vi "Load Command.vi"(8 "error in (no error)":errorcluster, 9 "Front (T) Back (F)":bool, 10 "Command In":refnum<class "Command.lvclass">, 11 "Command Handler in":refnum<class "Command Handler.lvclass">) -> (0 "error out":errorcluster, 3 "Command Handler out":refnum<class "Command Handler.lvclass">)   [LabVIEW 2017, in "Command Handler.lvlib" / "Command Handler.lvclass"]
uses:
  Command Handler.lvclass
  Command Parents/Command.lvclass
  Command Handler.lvclass/Command Handler.ctl
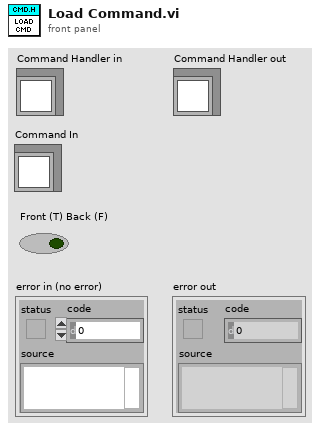
[diagram p1: front panel]
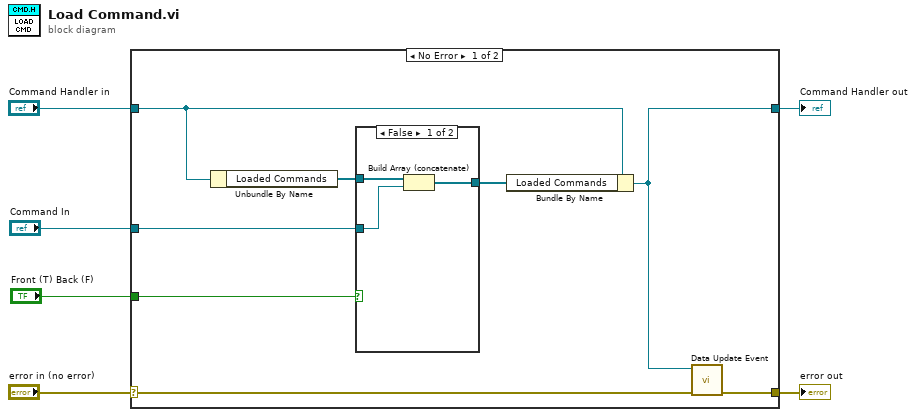
[diagram p0: block diagram]
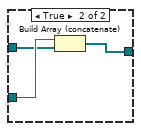
[diagram p2: hidden frame]
diagram:
  n1 = case shown="No Error" "error in (no error)" {
    selector: "error in (no error)" -> [w8 w22]
    tunnel: [w7 w22] -> w5
    tunnel: [w9 w21] -> w3
    tunnel: "Command Handler in" -> [w10 w21]
    tunnel: "Command In" -> [w13 _]
    tunnel: "Front (T) Back (F)" -> [w12 _]
    frame No Error {
      n2 = Unbundle By Name(w10) -> ("Loaded Commands"=w14:refnum<class "Command.lvclass">[])
      n3 = case shown="False" w12 {
        tunnel: w14 -> [w17 w19]
        tunnel: w13 -> [w16 w20]
        tunnel: [w15 w18] -> w11
        frame False {
          n4 = Build Array (concatenate)(w17, w16) -> (w15:refnum<class "Command.lvclass">[])
        }
        frame True {
          n5 = Build Array (concatenate)(w20, w19) -> (w18:refnum<class "Command.lvclass">[])
        }
      }
      n6 = Bundle By Name(cluster=w10, "Loaded Commands"=w11) -> (w9:refnum<class "Command Handler.lvclass">)
      n7 = call "Data Update Event.vi"("error in (no error)"=w8, "Command Handler in"=w9) -> ("error out"=w7:errorcluster)  [unwired: 9 in]
    }
    frame Error {
    }
  }
  "error out" <- w5
  "Command Handler out" <- w3
